vi "programa9.vi"() -> ()   [LabVIEW 2011]
panel:
  in  "on/off Prg":bool
  out "Temp minima":dbl
  out "Temop maxima":dbl
  out "Temp promedio":dbl
  in  "on/off A/C":bool
  out "A/C on":bool
  in  "Temp deseada":dbl
  out "Temperatura":i32(slide) scale=0.0..50.0
  # "el programa simula el funcionamiento de un a/c donde se ingresa la temperatura deseada y cada vez que la temperatura deseada \nsea mayor a temperatura no enciende el compresor del a/c pero cuando esta sea menor si enciende el compresor pero esto solo \npuede ocurrir siempre que el a/c este encendido, el programa termina solo cuando s=deicdimos nosotros terminar."
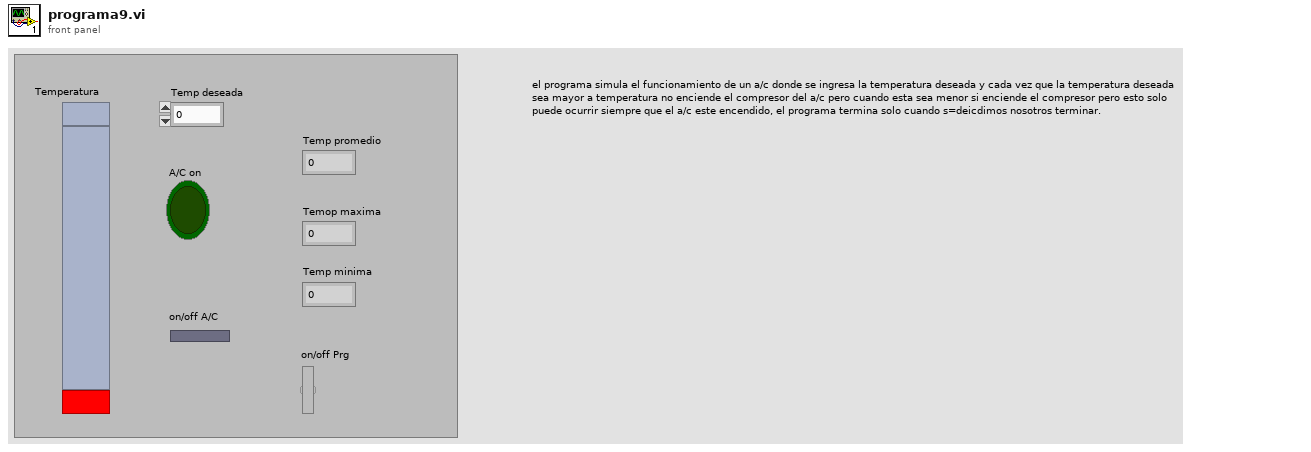
[diagram p1: front panel]
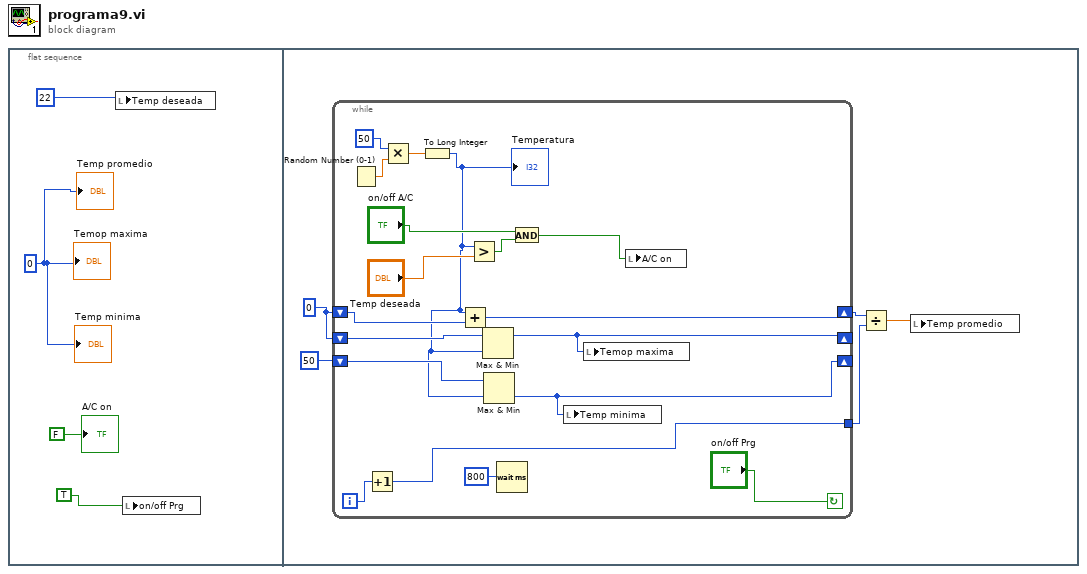
[diagram p0: block diagram]
diagram:
  n1 = flat-sequence {
    frame #0 {
      w4 = 0
      n2 = local write "Temp deseada"(22) -> ()
      n3 = local write "on/off Prg"(TRUE) -> ()
      "A/C on" <- FALSE
      "Temop maxima" <- w4
      "Temp minima" <- w4
      "Temp promedio" <- w4
    }
    frame #1 {
      w6 = 0
      n4 = while {
        shift-right: [w17] -> w9
        shift-left: w6 -> [w18]
        tunnel: [w15] -> w8
        shift-right: [w11] -> _
        shift-left: w6 -> [w14]
        shift-right: [w10] -> _
        shift-left: 50 -> [w13]
        i -> [w16]
        stop <- "on/off Prg" continue-if-true
        n5 = Random Number (0-1)() -> (number: 0 to 1=w26:dbl)
        n6 = Increment(x=w16) -> (x+1=w15:i32)
        n7 = Multiply(x=50, y=w26) -> (x*y=w27:dbl)
        n8 = To Long Integer(number=w27) -> (32bit integer=w12:i32)
        "Temperatura" <- w12
        n9 = Add(x=w12, y=w18) -> (x+y=w17:i32)
        n10 = Greater?(x=w12, y="Temp deseada") -> (0:w21:bool)
        n11 = Max & Min(x=w14, y=w12) -> (max(x,y)=w11:i32)  [unwired: 1 out]
        n12 = Max & Min(x=w13, y=w12) -> (min(x,y)=w10:i32)  [unwired: 1 out]
        n13 = Wait (ms)(milliseconds to wait=800) -> ()  [unwired: 1 out]
        n14 = And(x="on/off A/C", y=w21) -> (x .and. y?=w19:bool)
        n15 = local write "Temp minima"(w10) -> ()
        n16 = local write "Temop maxima"(w11) -> ()
        n17 = local write "A/C on"(w19) -> ()
      }
      n18 = Divide(x=w9, y=w8) -> (x/y=w7:dbl)
      n19 = local write "Temp promedio"(w7) -> ()
    }
  }
